vi "Message to Array - Test Results.vi"(0 "reference in":refnum<class "Result Logger.lvclass">, 4 "Messages":T1[](array[typedef]), 5 "error in (no error)":errorcluster) -> (14 "reference out":refnum<class "Result Logger.lvclass">, 18 "Array - Test Results":string[][](array[string]), 19 "error out":errorcluster)   [LabVIEW 2017, in "Result Logger.lvclass"]
uses:
  Result Logger.lvclass
  public/Message.ctl
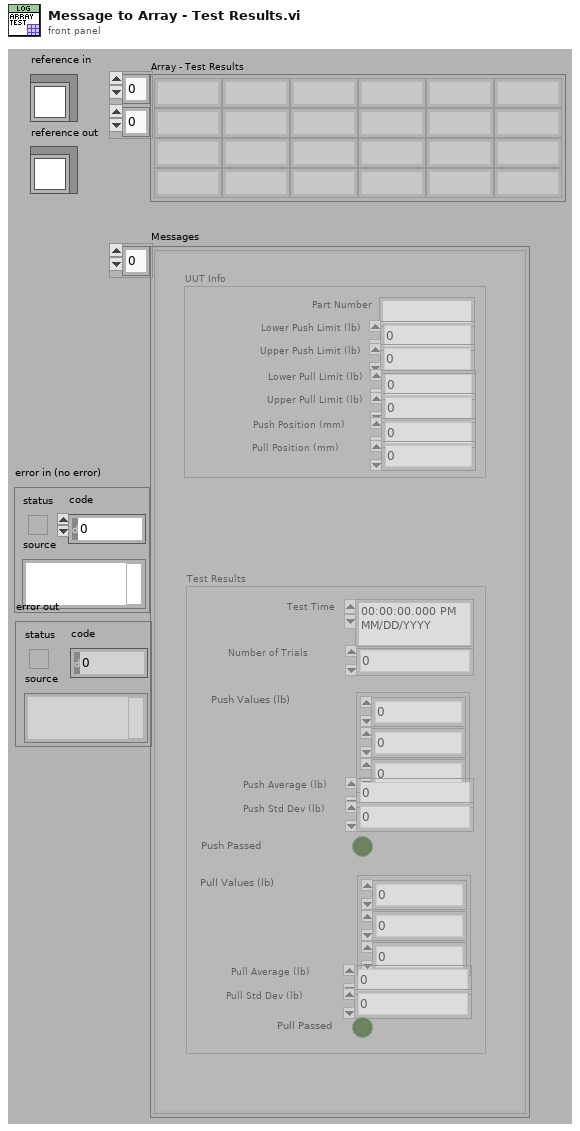
[diagram p1: front panel]
types:
  T1 = typedef "Result Logger.lvclass/Message.ctl" = cluster{"UUT Info":cluster{"Part Number":string, "Lower Push Limit (lb)":dbl, "Upper Push Limit (lb)":dbl, "Lower Pull Limit (lb)":dbl, "Upper Pull Limit (lb)":dbl, "Push Position (mm)":dbl, "Pull Position (mm)":dbl}, "Test Results":cluster{"Test Time":timestamp, "Number of Trials":u32, "Push Values (lb)":dbl[], "Push Average (lb)":dbl, "Push Std Dev (lb)":dbl, "Push Passed":bool, "Pull Values (lb)":dbl[], "Pull Average (lb)":dbl, "Pull Std Dev (lb)":dbl, "Pull Passed":bool}}
  T2 = cluster{"Part Number":string, "Lower Push Limit (lb)":dbl, "Upper Push Limit (lb)":dbl, "Lower Pull Limit (lb)":dbl, "Upper Pull Limit (lb)":dbl, "Push Position (mm)":dbl, "Pull Position (mm)":dbl}
  T3 = cluster{"Test Time":timestamp, "Number of Trials":u32, "Push Values (lb)":dbl[], "Push Average (lb)":dbl, "Push Std Dev (lb)":dbl, "Push Passed":bool, "Pull Values (lb)":dbl[], "Pull Average (lb)":dbl, "Pull Std Dev (lb)":dbl, "Pull Passed":bool}
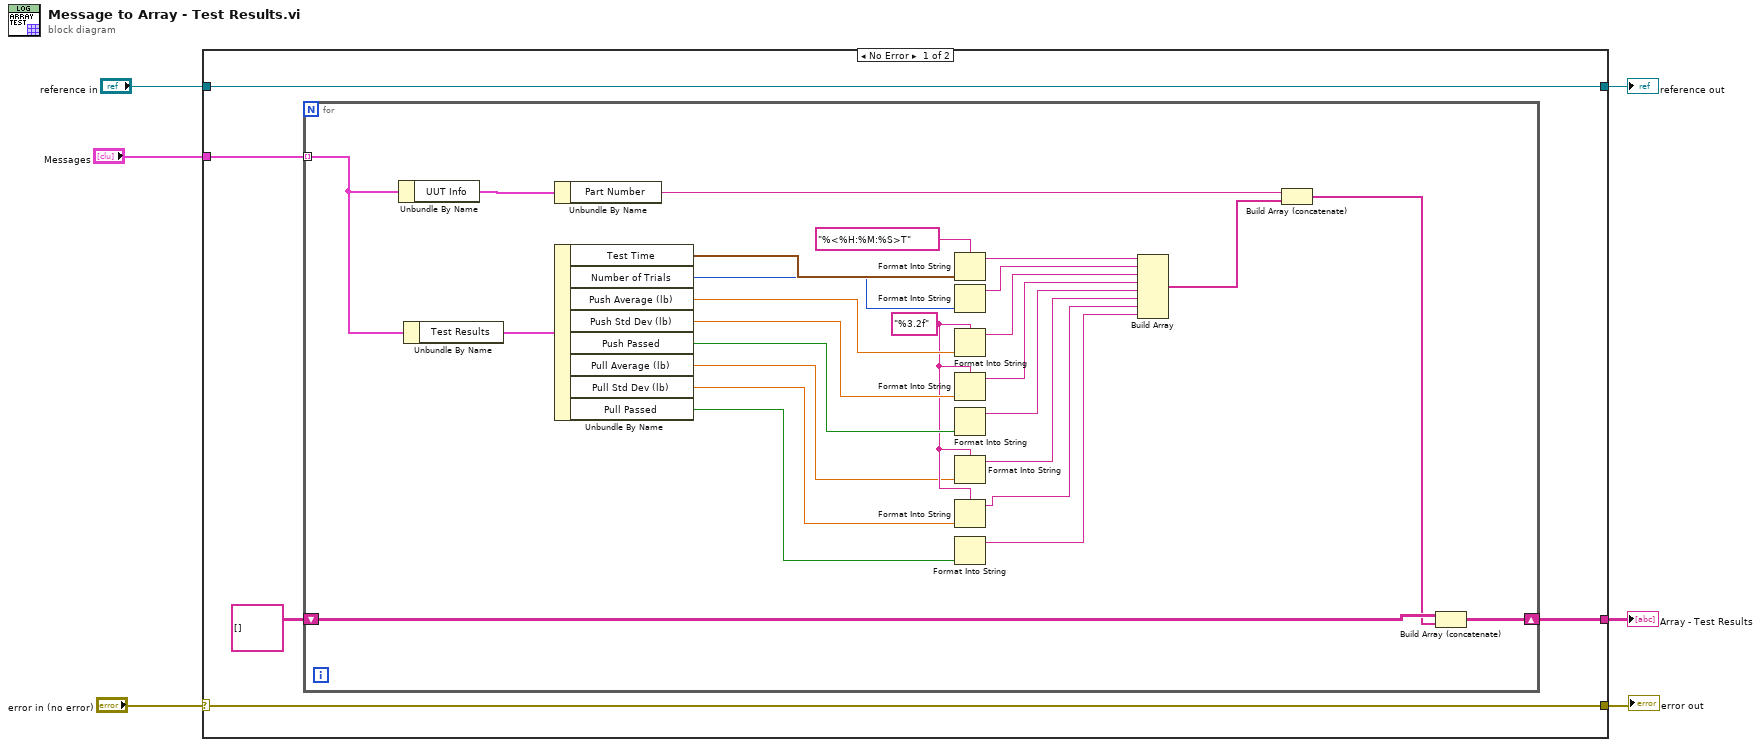
[diagram p0: block diagram]
diagram:
  n1 = case shown="No Error" "error in (no error)" {
    selector: "error in (no error)" -> [w10 w39]
    tunnel: [w10 w39] -> w5
    tunnel: [w11 w38] -> w3
    tunnel: "reference in" -> [w11 w38]
    tunnel: "Messages" -> [w9 _]
    tunnel: [w8 _] -> w2
    frame No Error {
      n2 = for {
        tunnel: w9 -> [w36] mode=indexing
        shift-right: [w13] -> w8
        shift-left: string[][] [] -> [w37]
        w27 = "%3.2f" ("format string")
        n3 = Unbundle By Name(w36) -> ("UUT Info"=w35:T2)
        n4 = Unbundle By Name(w36) -> ("Test Results"=w34:T3)
        n5 = Unbundle By Name(w35) -> ("Part Number"=w12:string)
        n6 = Unbundle By Name(w34) -> ("Test Time"=w32:timestamp, "Number of Trials"=w31:u32, "Push Average (lb)"=w30:dbl, "Push Std Dev (lb)"=w29:dbl, "Push Passed"=w28:bool, "Pull Average (lb)"=w26:dbl, "Pull Std Dev (lb)"=w25:dbl, "Pull Passed"=w24:bool)
        n7 = Format Into String(format string="%<%H:%M:%S>T", w32) -> (resulting string=w23:string)  [unwired: 2 in, 1 out]
        n8 = Format Into String(w31) -> (resulting string=w22:string)  [unwired: 3 in, 1 out]
        n9 = Format Into String(format string=w27, w30) -> (resulting string=w21:string)  [unwired: 2 in, 1 out]
        n10 = Format Into String(format string=w27, w29) -> (resulting string=w20:string)  [unwired: 2 in, 1 out]
        n11 = Format Into String(w28) -> (resulting string=w19:string)  [unwired: 3 in, 1 out]
        n12 = Format Into String(format string=w27, w26) -> (resulting string=w18:string)  [unwired: 2 in, 1 out]
        n13 = Format Into String(format string=w27, w25) -> (resulting string=w17:string)  [unwired: 2 in, 1 out]
        n14 = Format Into String(w24) -> (resulting string=w16:string)  [unwired: 3 in, 1 out]
        n15 = Build Array(w23, w22, w21, w20, w19, w18, w17, w16) -> (w15:string[])
        n16 = Build Array (concatenate)(w12, w15) -> (w14:string[])
        n17 = Build Array (concatenate)(w37, w14) -> (w13:string[][])
      }
    }
    frame Error {
    }
  }
  "error out" <- w5
  "reference out" <- w3
  "Array - Test Results" <- w2
